vi "ui get all files from folder recursively.vi"() -> ()   [LabVIEW 2023]
panel:
  out "size(s)":i32
  out "All Files in Dir":path[](array[path])
  in  "pattern (*.jpg)":string
  in  "Folder Path":path
  # "You can use the question mark character (?) to match any single character. You can use the asterisk character (*) to match any sequence of zero or more characters. For example, if you want this VI to find a list of the VIs in a folder, specify *.vi for pattern."
  # "Limited to one file type. Empty = all files"
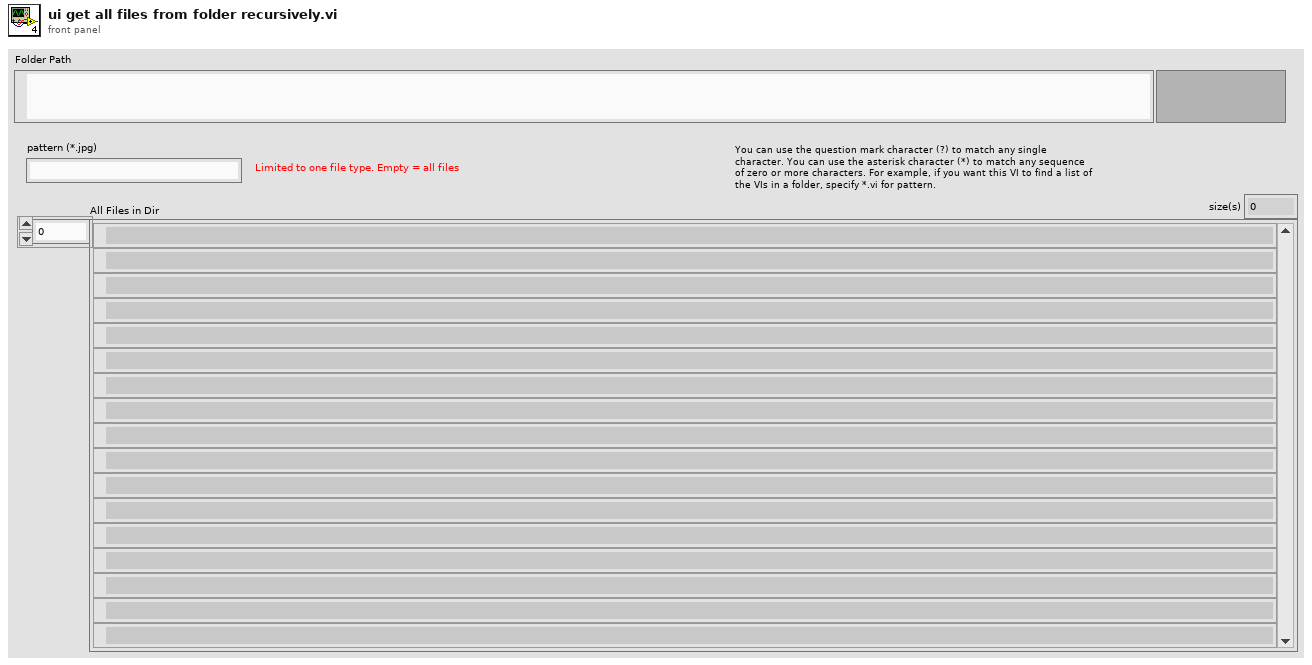
[diagram p1: front panel]
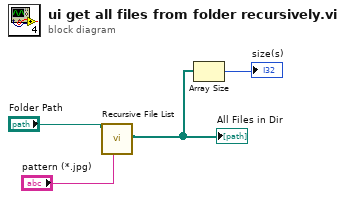
[diagram p0: block diagram]
diagram:
  n1 = call <vilib>:"Recursive File List.vi"("pattern"="pattern (*.jpg)", "Folder Path"="Folder Path") -> ("All Files in Dir"=w2:path[])  [unwired: 5 in, 4 out]
  "All Files in Dir" <- w2
  n2 = Array Size(array=w2) -> (size(s)=→"size(s)":i32)
